vi "CLD 8 CSV file commands utility Solution.vi"(8 "Fehler (Eingang)":T2) -> (0 "Fehler (Ausgang)":T2, 3 "Befehls-Ausgangs-Array":T1[](array[typedef]))   [LabVIEW 2009]
doc: "CLD 8 - Liest Daten aus einer CSV-Datei und fügt diese in ein Array aus Clustern ein."
uses:
  <vilib>/Utility/file.llb/Read From Spreadsheet File (string).vi
  CLD 8 Data Cluster.ctl
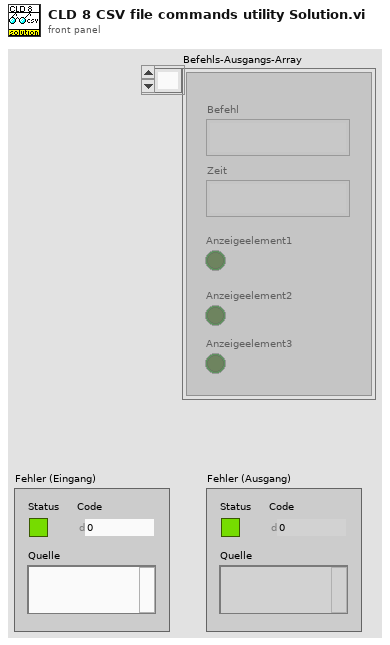
[diagram p1: front panel]
types:
  T1 = typedef "CLD 8 Data Cluster.ctl" = cluster{"Befehl":string, "Zeit":string, "Anzeigeelement1":bool, "Anzeigeelement2":bool, "Anzeigeelement3":bool}
  T2 = cluster{"Status":bool, "Code":i32, "Quelle":string}
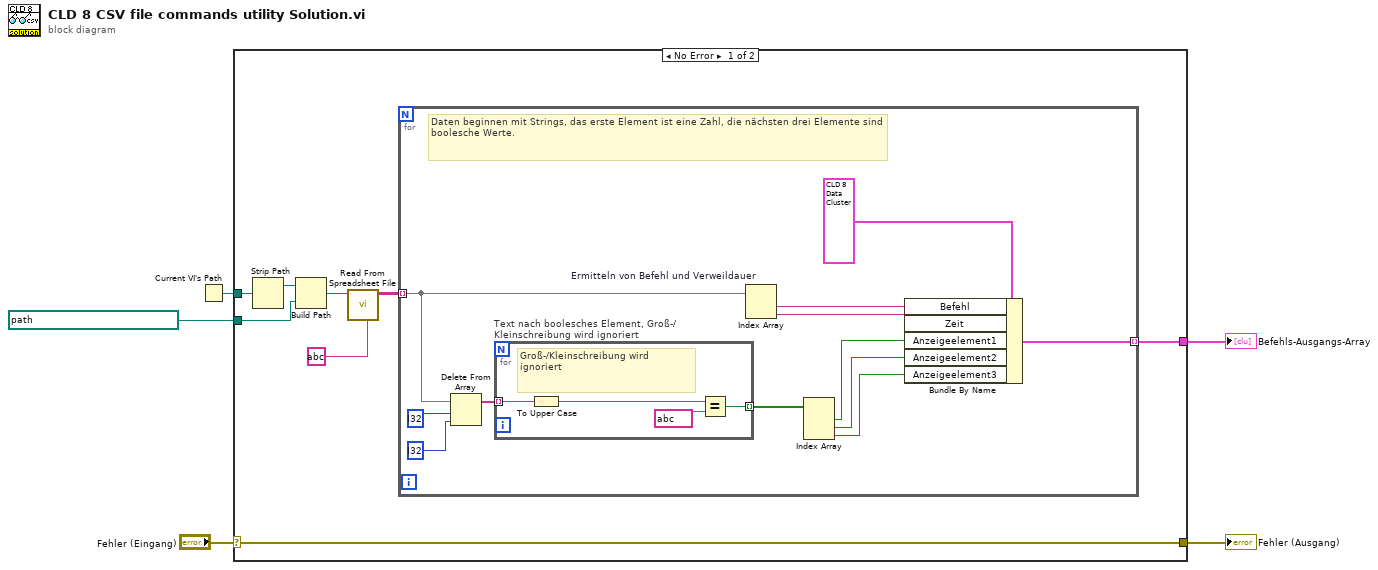
[diagram p0: block diagram]
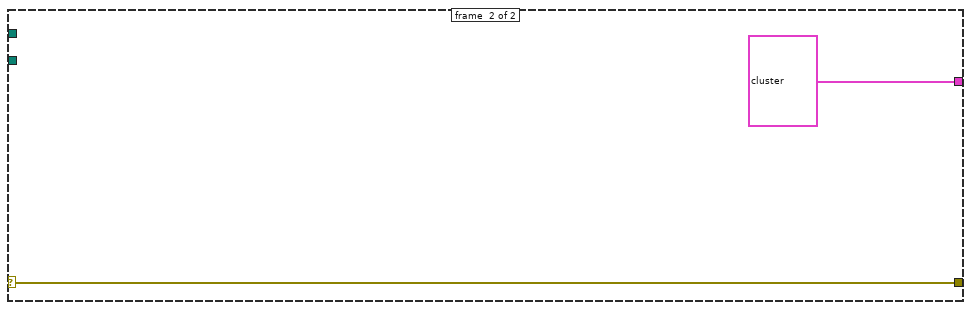
[diagram p2: hidden frame]
diagram:
  n1 = Current VI's Path() -> (path=w2:path)
  n2 = case shown="No Error" "Fehler (Eingang)" {
    selector: "Fehler (Eingang)" -> [w13 w31]
    tunnel: [w10 T1[] ?] -> w1
    tunnel: path ? -> [w8 _]
    tunnel: w2 -> [w9 _]
    tunnel: [w13 w31] -> w3
    frame #0 {
      n3 = Strip Path(path=w9) -> (stripped path=w6:path)  [unwired: 1 out]
      n4 = Build Path(base path=w6, name or relative path=w8) -> (appended path=w7:path)
      n5 = call-poly <vilib>:"Read From Spreadsheet File.vi"("delimiter (\\t)"=string ? ("Trennzeichen (\\t)"), "file path (dialog if empty)"=w7) -> ("all rows"=w12:string[][])  [unwired: 5 in, 4 out]
      n6 = for {
        tunnel: w12 -> [w25] mode=indexing
        tunnel: [w14] -> w10 mode=indexing
        # "Daten beginnen mit Strings, das erste Element ist eine Zahl, die nächsten drei Elemente sind boolesche Werte."
        n7 = Delete From Array(array=w25, length=i32 ? ("Länge"), index=i32 ? ("Index")) -> (array with subset deleted=w21:string[])  [unwired: 1 out]
        n8 = for "Text nach boolesches Element, Groß-/Kleinschreibung wird ignoriert" {
          tunnel: w21 -> [w29] mode=indexing
          tunnel: [w26] -> w22 mode=indexing
          # "Groß-/Kleinschreibung wird ignoriert"
          n9 = To Upper Case(1:w29) -> (0:w28:string)
          n10 = Equal?(x=w28, y=string ?) -> (x = y?=w26:bool)
        }
        n11 = Index Array "Ermitteln von Befehl und Verweildauer"(array=w25) -> (element #1=w19:string, element #2=w18:string)  [unwired: 2 in]
        n12 = Index Array(array=w22) -> (element #1=w17:bool, element #2=w16:bool, element #3=w15:bool)  [unwired: 3 in]
        n13 = Bundle By Name(cluster=T1 ? ("Cluster 3"), "Befehl"=w19, "Zeit"=w18, "Anzeigeelement1"=w17, "Anzeigeelement2"=w16, "Anzeigeelement3"=w15) -> (w14:T1)
      }
    }
    frame #1 {
    }
  }
  "Fehler (Ausgang)" <- w3
  "Befehls-Ausgangs-Array" <- w1
